vi "Teleop.vi"(0 "Call Context":T10) -> (6 "SubState 3":T1, 8 "SubState 4":T1, 9 "SubState 5":T9, 11 "Loop 3 Data":T5, 13 "Loop 4 Data":T4, 14 "SubState 0":T1=enum."driver control", 15 "Loop 1 Data":T7, 16 "Loop 0 Data":T8, 17 "SubState 1":T1, 18 "Loop 2 Data":T6, 19 "SubState 2":T1)   [LabVIEW 2013]
uses:
  typedefs/subStates.ctl
  <vilib>/Rock Robotics/WPI/DriverStation/WPI_DriverStationDerivedRobotMode.ctl
  typedefs/singleUseSubstate.ctl
  typedefs/Loop Datatypes/Loop 0 Datatype.ctl
  typedefs/Loop Datatypes/Loop 1 Datatype.ctl
  typedefs/Loop Datatypes/Loop 2 Datatype.ctl
  typedefs/Loop Datatypes/Loop 3 Datatype.ctl
  typedefs/Loop Datatypes/Loop 4 Datatype.ctl
  <vilib>/Rock Robotics/WPI/Joystick/WPI_JoystickDevRef.ctl
  <vilib>/Rock Robotics/WPI/Joystick/WPI_JoystickDeviceEnum.ctl
  typedefs/fg_typedef.ctl
  typedefs/vision enable.ctl
  <vilib>/Rock Robotics/WPI/Joystick/WPI_JoystickGetSetRefNum.vi
panel:
  out "prev lock state":T1
  out "JS3":T2
  out "Drive to DC":bool
  out "JS1":T2
  out "JS2":T2
  out "Exit Value":i32=-1
  # "Loop Data and Substates"
  # "Latch Loop"
  # "Drive Loop"
  # "Shooter Pneumatics Loop"
  # "Pickup/Passing Belts Loop"
  # "Pickup Arm Loop"
  # "Shifter Loop"
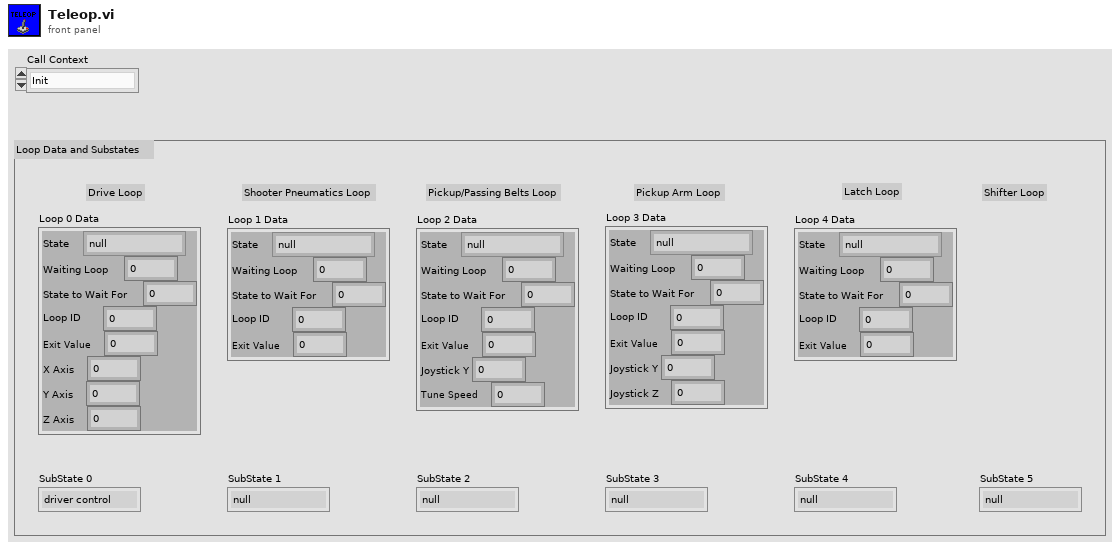
[diagram p1: front panel]
types:
  T1 = typedef "subStates.ctl" = enum16{"null", "wait", "driver control", "auto", "manual override", "hold position", "rotate", "pickup", "pass", "load", "goto shoot", "shoot", "cancel", "end"}
  T2 = typedef "WPI_JoystickDevRef.ctl" = cluster{"Device":T3}
  T3 = typedef "WPI_JoystickDeviceEnum.ctl" = enum16{"USB 1", "USB 2", "USB 3", "USB 4", "Kinect 1", "Kinect 2"}
  T4 = typedef "Loop 4 Datatype.ctl" = cluster{"State":T1, "Waiting Loop":i32, "State to Wait For":i32, "Loop ID":i32, "Exit Value":i32}
  T5 = typedef "Loop 3 Datatype.ctl" = cluster{"State":T1, "Waiting Loop":i32, "State to Wait For":i32, "Loop ID":i32, "Exit Value":i32, "Joystick Y":dbl, "Joystick Z":dbl}
  T6 = typedef "Loop 2 Datatype.ctl" = cluster{"State":T1, "Waiting Loop":i32, "State to Wait For":i32, "Loop ID":i32, "Exit Value":i32, "Joystick Y":dbl, "Tune Speed":dbl}
  T7 = typedef "Loop 1 Datatype.ctl" = cluster{"State":T1, "Waiting Loop":i32, "State to Wait For":i32, "Loop ID":i32, "Exit Value":i32}
  T8 = typedef "Loop 0 Datatype.ctl" = cluster{"State":T1, "Waiting Loop":i32, "State to Wait For":i32, "Loop ID":i32, "Exit Value":i32, "X Axis":dbl, "Y Axis":dbl, "Z Axis":dbl}
  T9 = typedef "singleUseSubstate.ctl" = enum16{"null", "wait", "shift high", "shift low"}
  T10 = typedef "WPI_DriverStationDerivedRobotMode.ctl" = enum16{"Init", "Execute", "Stop"}
  T11 = cluster{"axis 1 (x)":dbl, "axis 2 (y)":dbl, "axis 3 (throttle)":dbl, "axis 4":dbl, "axis 5":dbl, "axis 6":dbl}
  T12 = typedef "WPI_EncoderDevRef.ctl" = cluster{"DevStatus":errorcluster, "EncoderIndex":T13, "CounterIndex":T14, "DistancePerCount":dbl, "Decoding Type":T15}
  T13 = typedef "FPGA_EncoderIdx.ctl" = enum8{"Enc 0", "Enc 1", "Enc 2", "Enc 3", "Invalid"}
  T14 = typedef "FPGA_CounterCtrSystemIndex.ctl" = enum8{"Ctr 0", "Ctr 1", "Ctr 2", "Ctr 3", "Ctr 4", "Ctr 5", "Ctr 6", "Ctr 7", "Invalid"}
  T15 = typedef "WPI_EncoderType.ctl" = enum16{"1x", "2x", "4x"}
  T16 = typedef "vision enable.ctl" = enum16{"Enable", "Disable", "Stop"}
  T17 = typedef "fg_typedef.ctl" = enum16{"Get", "Set"}
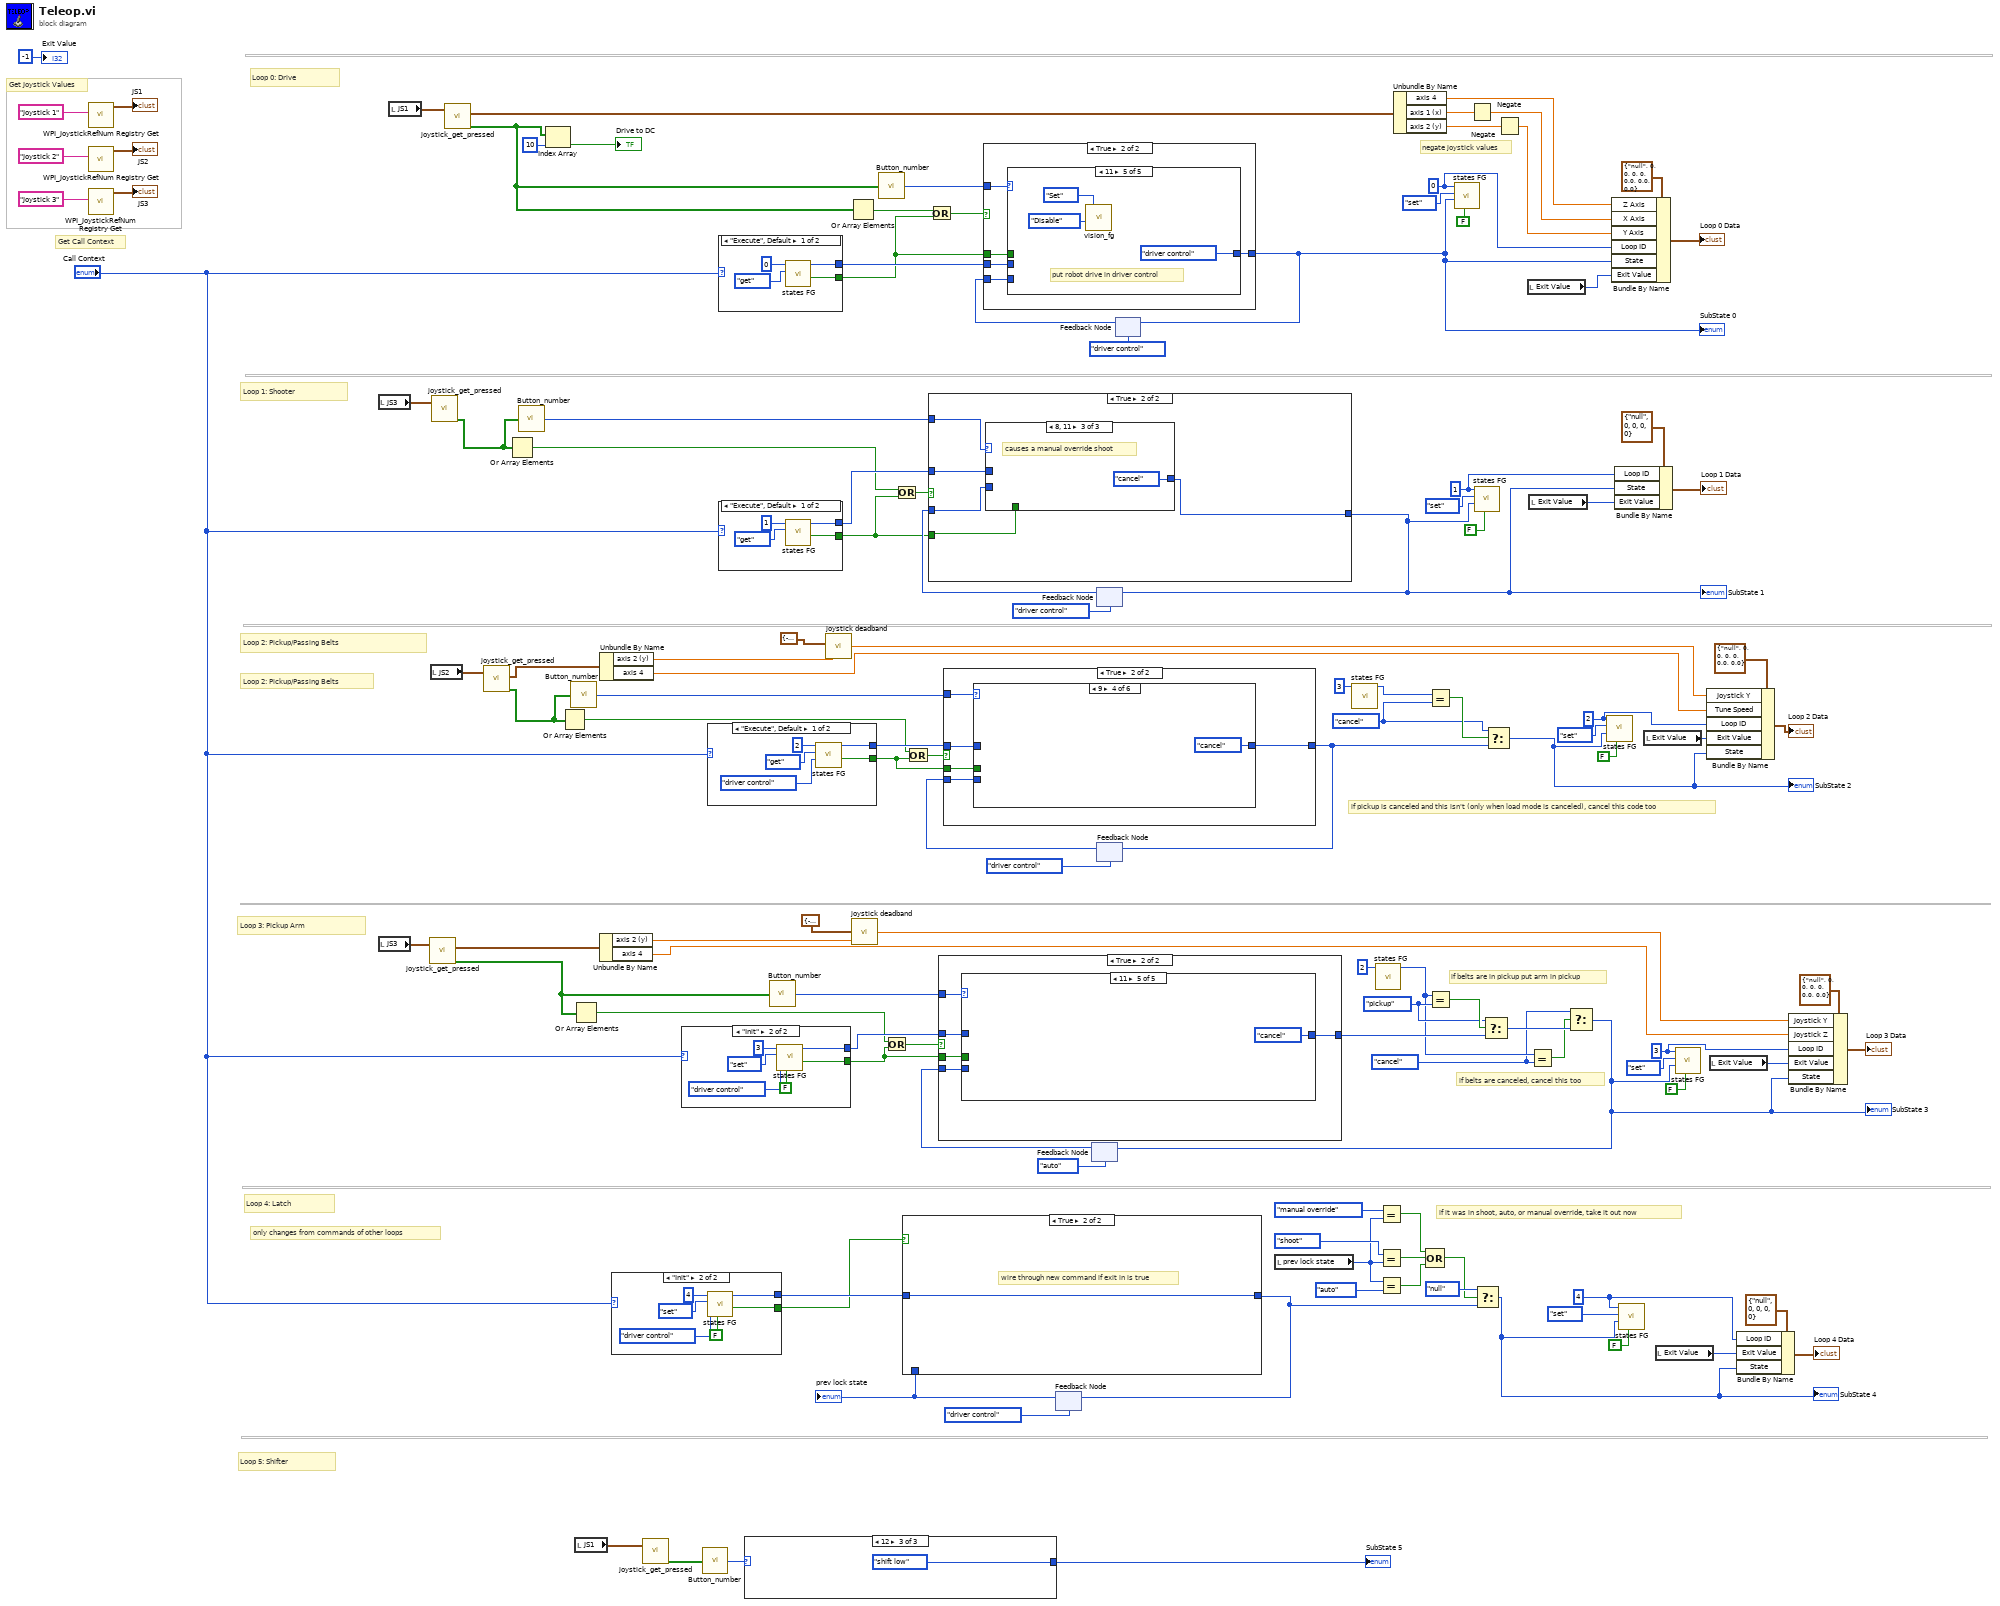
[diagram p0: block diagram]
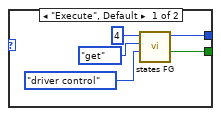
[diagram p3: hidden frame]
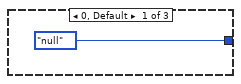
[diagram p4: hidden frame]
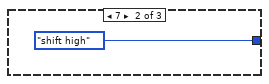
[diagram p5: hidden frame]
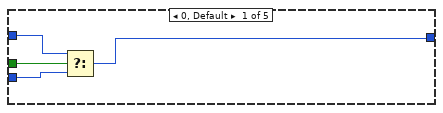
[diagram p7: hidden frame]
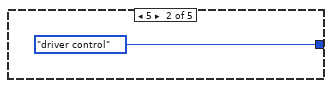
[diagram p8: hidden frame]
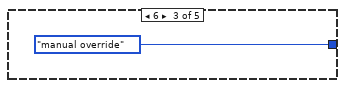
[diagram p9: hidden frame]
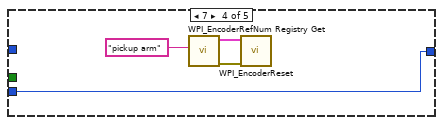
[diagram p10: hidden frame]
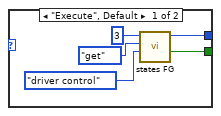
[diagram p11: hidden frame]
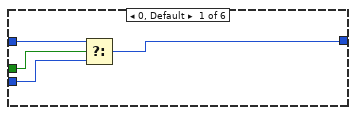
[diagram p13: hidden frame]
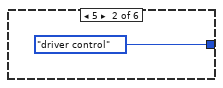
[diagram p14: hidden frame]
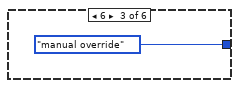
[diagram p15: hidden frame]
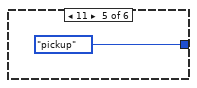
[diagram p16: hidden frame]
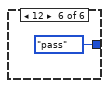
[diagram p17: hidden frame]
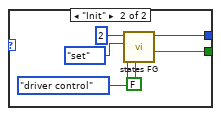
[diagram p18: hidden frame]
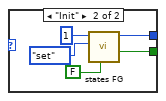
[diagram p19: hidden frame]
diagram:
  w1 = subStates."cancel" ("y")
  w8 = subStates."cancel" ("y")
  w25 = subStates."pickup" ("y")
  w36 = 4 ("Loop ID")
  w100 = 3 ("Loop ID")
  w101 = 2 ("Loop ID")
  w110 = 1 ("Loop ID")
  w112 = 0 ("Loop ID")
  # "if pickup is canceled and this isn't (only when load mode is canceled), cancel this code too"
  # "if belts are canceled, cancel this too"
  # "only changes from commands of other loops"
  # "if it was in shoot, auto, or manual override, take it out now"
  # "if belts are in pickup put arm in pickup"
  # "Loop 2: Pickup/Passing Belts"
  # "negate joystick values"
  # "Get Call Context"
  # "Get Joystick Values"
  # "Loop 4: Latch"
  # "Loop 3: Pickup Arm"
  # "Loop 5: Shifter"
  # "Loop 2: Pickup/Passing Belts"
  # "Loop 1: Shooter"
  # "Loop 0: Drive"
  n1 = call <vilib>:"WPI_JoystickRefNum Registry Get.vi"("refnum name"="Joystick 1") -> ("JoystickDevRef"=→"JS1":T2)  [unwired: 9 in, 1 out]
  n2 = call <vilib>:"WPI_JoystickRefNum Registry Get.vi"("refnum name"="Joystick 2") -> ("JoystickDevRef"=→"JS2":T2)  [unwired: 9 in, 1 out]
  n3 = call <vilib>:"WPI_JoystickRefNum Registry Get.vi"("refnum name"="Joystick 3") -> ("JoystickDevRef"=→"JS3":T2)  [unwired: 9 in, 1 out]
  n4 = local read "JS3"() -> (w77:T2)
  n5 = local read "JS3"() -> (w62:T2)
  n6 = local read "JS1"() -> (w78:T2)
  n7 = call "joystick_get_pressed.vi"("JoystickDevRef 2"=w62) -> ("Axes"=w66:T11, "Buttons Pressed?"=w43:bool[])  [unwired: 1 in, 2 out]
  n8 = local read "JS2"() -> (w50:T2)
  n9 = call "joystick_get_pressed.vi"("JoystickDevRef 2"=w77) -> ("Buttons Pressed?"=w45:bool[])  [unwired: 1 in, 3 out]
  n10 = call "joystick_get_pressed.vi"("JoystickDevRef 2"=w78) -> ("Axes"=w82:T11, "Buttons Pressed?"=w58:bool[])  [unwired: 1 in, 2 out]
  n11 = call "joystick_get_pressed.vi"("JoystickDevRef 2"=w50) -> ("Axes"=w33:T11, "Buttons Pressed?"=w34:bool[])  [unwired: 1 in, 2 out]
  n12 = Or Array Elements(Boolean array=w45) -> (logical OR=w69:bool)
  n13 = call "Button_number.vi"("Button Array"=w45) -> ("Button Pressed"=w71:i32)
  n14 = Index Array(array=w58, index=10) -> (element=→"Drive to DC":bool)
  n15 = Or Array Elements(Boolean array=w34) -> (logical OR=w49:bool)
  n16 = call "Button_number.vi"("Button Array"=w34) -> ("Button Pressed"=w48:i32)
  n17 = Or Array Elements(Boolean array=w43) -> (logical OR=w65:bool)
  n18 = local read "JS1"() -> (w53:T2)
  n19 = Unbundle By Name(w66) -> ("axis 2 (y)"=w61:dbl, "axis 4"=w29:dbl)
  n20 = Unbundle By Name(w33) -> ("axis 2 (y)"=w42:dbl, "axis 4"=w31:dbl)
  n21 = case shown="\"Init\"" "Call Context" {
    tunnel: [w131 w137] -> w13
    tunnel: [w129 w134] -> w38
    frame "Execute", Default {
      n22 = call "states FG.vi"("subState in"=subStates."driver control", "menu (get)"=enum16{"set", "get"}."get", "Loop ID"=4) -> ("exit out"=w131:bool, "subState out"=w129:T1)  [unwired: 5 in, 2 out]
    }
    frame "Init" {
      n23 = call "states FG.vi"("exit in"=FALSE, "subState in"=subStates."driver control", "menu (get)"=enum16{"set", "get"}."set", "Loop ID"=4) -> ("exit out"=w137:bool, "subState out"=w134:T1)  [unwired: 4 in, 2 out]
    }
  }
  n24 = call "joystick_get_pressed.vi"("JoystickDevRef 2"=w53) -> ("Buttons Pressed?"=w55:bool[])  [unwired: 1 in, 3 out]
  n25 = case shown="\"Init\"" "Call Context" {
    tunnel: [w142 w148] -> w63
    tunnel: [w140 w145] -> w98
    frame "Execute", Default {
      n26 = call "states FG.vi"("subState in"=subStates."driver control", "menu (get)"=enum16{"set", "get"}."get", "Loop ID"=3) -> ("exit out"=w142:bool, "subState out"=w140:T1)  [unwired: 5 in, 2 out]
    }
    frame "Init" {
      n27 = call "states FG.vi"("exit in"=FALSE, "subState in"=subStates."driver control", "menu (get)"=enum16{"set", "get"}."set", "Loop ID"=3) -> ("exit out"=w148:bool, "subState out"=w145:T1)  [unwired: 4 in, 2 out]
    }
  }
  n28 = call "Button_number.vi"("Button Array"=w55) -> ("Button Pressed"=w54:i32)
  n29 = case shown="\"Execute\", Default" "Call Context" {
    tunnel: [w153 w159] -> w68
    tunnel: [w151 w156] -> w117
    frame "Execute", Default {
      n30 = call "states FG.vi"("subState in"=subStates."driver control", "menu (get)"=enum16{"set", "get"}."get", "Loop ID"=2) -> ("exit out"=w153:bool, "subState out"=w151:T1)  [unwired: 5 in, 2 out]
    }
    frame "Init" {
      n31 = call "states FG.vi"("exit in"=FALSE, "subState in"=subStates."driver control", "menu (get)"=enum16{"set", "get"}."set", "Loop ID"=2) -> ("exit out"=w159:bool, "subState out"=w156:T1)  [unwired: 4 in, 2 out]
    }
  }
  n32 = case shown="\"Execute\", Default" "Call Context" {
    tunnel: [w163 w168] -> w75
    tunnel: [w162 w166] -> w115
    frame "Execute", Default {
      n33 = call "states FG.vi"("menu (get)"=enum16{"set", "get"}."get", "Loop ID"=0) -> ("exit out"=w163:bool, "subState out"=w162:T1)  [unwired: 6 in, 2 out]
    }
    frame "Init" {
      n34 = call "states FG.vi"("exit in"=FALSE, "menu (get)"=enum16{"set", "get"}."set", "Loop ID"=0) -> ("exit out"=w168:bool, "subState out"=w166:T1)  [unwired: 5 in, 2 out]
    }
  }
  n35 = case shown="\"Execute\", Default" "Call Context" {
    tunnel: [w172 w177] -> w72
    tunnel: [w171 w175] -> w114
    frame "Execute", Default {
      n36 = call "states FG.vi"("menu (get)"=enum16{"set", "get"}."get", "Loop ID"=1) -> ("exit out"=w172:bool, "subState out"=w171:T1)  [unwired: 6 in, 2 out]
    }
    frame "Init" {
      n37 = call "states FG.vi"("exit in"=FALSE, "menu (get)"=enum16{"set", "get"}."set", "Loop ID"=1) -> ("exit out"=w177:bool, "subState out"=w175:T1)  [unwired: 5 in, 2 out]
    }
  }
  n38 = case shown="12" w54 {
    tunnel: [singleUseSubstate."null" ("Enum") singleUseSubstate."shift high" ("Enum") singleUseSubstate."shift low" ("Enum")] -> w90
    frame 0, Default {
    }
    frame 7 {
    }
    frame 12 {
    }
  }
  "SubState 5" <- w90
  n39 = call "Button_number.vi"("Button Array"=w43) -> ("Button Pressed"=w64:i32)
  n40 = call "joystick deadband.vi"("Joystick In"=w42, "Deadband Range"=cluster{"Deadband Min":dbl, "Deadband Max":dbl} {"Deadband Min"=-0.05, "Deadband Max"=0.05}) -> ("Joystick Out"=w32:dbl)  [unwired: 4 in]
  n41 = Or Array Elements(Boolean array=w58) -> (logical OR=w76:bool)
  n42 = call "joystick deadband.vi"("Joystick In"=w61, "Deadband Range"=cluster{"Deadband Min":dbl, "Deadband Max":dbl} {"Deadband Min"=-0.05, "Deadband Max"=0.05}) -> ("Joystick Out"=w30:dbl)  [unwired: 4 in]
  n43 = call "Button_number.vi"("Button Array"=w58) -> ("Button Pressed"=w81:i32)
  n44 = Or(x=w65, y=w63) -> (x .or. y?=w67:bool)
  n45 = Or(x=w69, y=w72) -> (x .or. y?=w73:bool)
  n46 = Or(x=w49, y=w68) -> (x .or. y?=w70:bool)
  n47 = Or(x=w76, y=w75) -> (x .or. y?=w74:bool)
  n48 = feedback #1(subStates."driver control" ("Drive SubState")) -> (w12:T1)
  "prev lock state" <- w12
  n49 = case shown="True" w13 {
    tunnel: [w183 w184] -> w23
    tunnel: w38 -> [_ w184]
    tunnel: w12 -> [w183 _]
    frame False {
      # "*yawn* nothing to do...wire through the previous state"
    }
    frame True {
      # "wire through new command if exit in is true"
    }
  }
  n50 = feedback-in #1(w23) -> ()
  n51 = feedback #2(subStates."auto" ("Drive SubState")) -> (w95:T1)
  n52 = case shown="True" w67 {
    tunnel: w95 -> [w185 w186]
    tunnel: [w185 w187] -> w27
    tunnel: w98 -> [_ w188]
    tunnel: w64 -> [_ w190]
    tunnel: w63 -> [_ w189]
    frame False {
      # "boring drivers, not pressing anything...wire through the previous state"
    }
    frame True {
      n53 = case shown="11" w190 {
        tunnel: w189 -> [w194 _ _ _ _]
        tunnel: w186 -> [w193 _ _ w200 _]
        tunnel: w188 -> [w192 _ _ _ _]
        tunnel: [w191 subStates."driver control" ("Drive SubState") subStates."manual override" ("Drive SubState") w200 subStates."cancel" ("Drive SubState")] -> w187
        frame 0, Default {
          n54 = Select(t=w192, s=w194, f=w193) -> (s? t:f=w191:T1)
        }
        frame 5 {
        }
        frame 6 {
        }
        frame 7 {
          n55 = call <vilib>:"WPI_EncoderRefNum Registry Get.vi"("refnum name"="pickup arm") -> ("error out"=w198:errorcluster, "EncoderDevRef"=w197:T12)  [unwired: 9 in]
          n56 = call <vilib>:"WPI_EncoderReset.vi"("error in (no error)"=w198, "EncoderDevRef"=w197) -> ()  [unwired: 8 in, 2 out]
        }
        frame 11 {
        }
      }
    }
  }
  n57 = feedback #3(subStates."driver control" ("Drive SubState")) -> (w116:T1)
  n58 = case shown="True" w73 {
    tunnel: w116 -> [w202 w206]
    tunnel: [w202 w203] -> w83
    tunnel: w114 -> [_ w207]
    tunnel: w71 -> [_ w205]
    tunnel: w72 -> [_ w204]
    frame False {
      # "nothing pressed here, move along (wire through the previous state)"
    }
    frame True {
      n59 = case shown="8, 11" w205 {
        tunnel: w207 -> [w210 _ _]
        tunnel: w206 -> [w209 _ _]
        tunnel: [w208 subStates."load" ("Drive SubState") subStates."cancel" ("Drive SubState")] -> w203
        tunnel: w204 -> [w211 _ _]
        frame 0, Default {
          n60 = Select(t=w210, s=w211, f=w209) -> (s? t:f=w208:T1)
        }
        frame 2 {
        }
        frame 8, 11 {
          # "causes a manual override shoot"
        }
      }
    }
  }
  "SubState 1" <- w83
  n61 = feedback-in #3(w83) -> ()
  n62 = feedback #4(subStates."driver control" ("Drive SubState")) -> (w120:T1)
  n63 = case shown="True" w70 {
    tunnel: w120 -> [w214 w216]
    tunnel: [w214 w215] -> w4
    tunnel: w117 -> [_ w217]
    tunnel: w48 -> [_ w219]
    tunnel: w68 -> [_ w218]
    frame False {
      # "nothing pressed here, move along obviously and wire through the previous state"
    }
    frame True {
      n64 = case shown="9" w219 {
        tunnel: w218 -> [w223 _ _ _ _ _]
        tunnel: w217 -> [w222 _ _ _ _ _]
        tunnel: w216 -> [w221 _ _ _ _ _]
        tunnel: [w220 subStates."driver control" ("Drive SubState") subStates."manual override" ("Drive SubState") subStates."cancel" ("Drive SubState") subStates."pickup" ("Drive SubState") subStates."pass" ("Drive SubState")] -> w215
        frame 0, Default {
          n65 = Select(t=w222, s=w223, f=w221) -> (s? t:f=w220:T1)
        }
        frame 5 {
        }
        frame 6 {
        }
        frame 9 {
        }
        frame 11 {
        }
        frame 12 {
        }
      }
    }
  }
  n66 = feedback-in #4(w4) -> ()
  n67 = feedback #5(subStates."driver control" ("Drive SubState")) -> (w122:T1)
  n68 = case shown="True" w74 {
    tunnel: w122 -> [w229 w231]
    tunnel: [w229 w230] -> w52
    tunnel: w115 -> [_ w232]
    tunnel: w81 -> [_ w234]
    tunnel: w75 -> [_ w233]
    frame False {
      # "keep current state, no change necessary"
    }
    frame True {
      n69 = case shown="11" w234 {
        tunnel: w233 -> [w238 _ _ _ _]
        tunnel: w232 -> [w237 _ _ _ _]
        tunnel: w231 -> [w236 w243 w244 w252 _]
        tunnel: [w235 w239 w244 w253 subStates."driver control" ("Drive SubState")] -> w230
        frame 0, Default {
          n70 = Select(t=w237, s=w238, f=w236) -> (s? t:f=w235:T1)
        }
        frame 1 {
          w240 = subStates."hold position" ("x")
          # "button 1, hold position toggle"
          n71 = Equal?(x=w240, y=w243) -> (x = y?=w242:bool)
          n72 = Select(t=subStates."driver control" ("Drive SubState"), s=w242, f=w240) -> (s? t:f=w239:T1)
        }
        frame 8 {
          n73 = disable-structure shown="Enabled" {
            frame Disabled {
              w247 = vision_enable."Enable" ("y")
              # "toggle vision"
              n74 = call "vision_fg.vi"("Menu"=fg_typedef."Get") -> ("State Out"=w249:T16)  [unwired: 2 in, 1 out]
              n75 = Equal?(x=w249, y=w247) -> (x = y?=w248:bool)
              n76 = Select(t=vision_enable."Disable" ("y"), s=w248, f=w247) -> (s? t:f=w245:T16)
              n77 = call "vision_fg.vi"("Action"=w245, "Menu"=fg_typedef."Set") -> ()  [unwired: 1 in, 2 out]
            }
            frame Enabled {
              # "no vision at suffield"
            }
          }
        }
        frame 9 {
          n78 = disable-structure shown="Enabled" {
            disable-tunnel: [subStates."goto shoot" ("Drive SubState") w257] -> w253
            disable-tunnel: w252 -> [_ w257]
            frame Disabled {
              # "go to shoot location"
              n79 = call "vision_fg.vi"("Action"=vision_enable."Enable", "Menu"=fg_typedef."Set") -> ()  [unwired: 1 in, 2 out]
            }
            frame Enabled {
              # "no vision at suffield"
            }
          }
        }
        frame 11 {
          # "put robot drive in driver control"
          n80 = call "vision_fg.vi"("Action"=vision_enable."Disable", "Menu"=fg_typedef."Set") -> ()  [unwired: 1 in, 2 out]
        }
      }
    }
  }
  "SubState 0" <- w52
  n81 = feedback-in #5(w52) -> ()
  n82 = local read "prev lock state"() -> (w19:T1)
  n83 = call "states FG.vi"("Loop ID"=3) -> ("subState out"=w5:T1)  [unwired: 7 in, 3 out]
  n84 = call "states FG.vi"("Loop ID"=2) -> ("subState out"=w11:T1)  [unwired: 7 in, 3 out]
  n85 = Equal?(x=subStates."manual override", y=w19) -> (x = y?=w17:bool)
  n86 = Equal?(x=subStates."shoot", y=w19) -> (x = y?=w16:bool)
  n87 = Equal?(x=w19, y=subStates."auto") -> (x = y?=w15:bool)
  n88 = Unbundle By Name(w82) -> ("axis 4"=w59:dbl, "axis 1 (x)"=w87:dbl, "axis 2 (y)"=w86:dbl)
  n89 = Compound Arithmetic op=OR(w17, w16, w15) -> (w14:bool)
  n90 = Equal?(x=w5, y=w1) -> (x = y?=w3:bool)
  n91 = Equal?(x=w11, y=w25) -> (x = y?=w26:bool)
  n92 = call "states FG.vi"("exit in"=FALSE, "subState in"=w52, "menu (get)"=enum16{"set", "get"}."set", "Loop ID"=w112) -> ()  [unwired: 4 in, 4 out]
  n93 = Negate(x=w87) -> (-x=w85:dbl)
  n94 = call "states FG.vi"("exit in"=FALSE, "subState in"=w83, "menu (get)"=enum16{"set", "get"}."set", "Loop ID"=w110) -> ()  [unwired: 4 in, 4 out]
  n95 = Select(t=subStates."null", s=w14, f=w23) -> (s? t:f=w22:T1)
  "SubState 4" <- w22
  n96 = Select(t=w25, s=w26, f=w27) -> (s? t:f=w10:T1)
  n97 = Select(t=w1, s=w3, f=w4) -> (s? t:f=w2:T1)
  "SubState 2" <- w2
  n98 = Negate(x=w86) -> (-x=w84:dbl)
  n99 = local read "Exit Value"() -> (w108:i32)
  n100 = local read "Exit Value"() -> (w107:i32)
  n101 = Equal?(x=w11, y=w8) -> (x = y?=w9:bool)
  n102 = Select(t=w8, s=w9, f=w10) -> (s? t:f=w7:T1)
  "SubState 3" <- w7
  n103 = feedback-in #2(w7) -> ()
  n104 = call "states FG.vi"("exit in"=FALSE, "subState in"=w2, "menu (get)"=enum16{"set", "get"}."set", "Loop ID"=w101) -> ()  [unwired: 4 in, 4 out]
  n105 = Bundle By Name(cluster=T8 {"State"=enum."null", "Waiting Loop"=0, "State to Wait For"=0, "Loop ID"=0, "Exit Value"=0, "X Axis"=0.0, "Y Axis"=0.0, "Z Axis"=0.0} ("Cluster"), "Z Axis"=w59, "X Axis"=w85, "Y Axis"=w84, "Loop ID"=w112, "State"=w52, "Exit Value"=w108) -> (→"Loop 0 Data":T8)
  n106 = Bundle By Name(cluster=T7 {"State"=enum."null", "Waiting Loop"=0, "State to Wait For"=0, "Loop ID"=0, "Exit Value"=0} ("Cluster"), "Loop ID"=w110, "State"=w83, "Exit Value"=w107) -> (→"Loop 1 Data":T7)
  n107 = call "states FG.vi"("exit in"=FALSE, "subState in"=w22, "menu (get)"=enum16{"set", "get"}."set", "Loop ID"=w36) -> ()  [unwired: 4 in, 4 out]
  n108 = local read "Exit Value"() -> (w102:i32)
  n109 = local read "Exit Value"() -> (w37:i32)
  n110 = call "states FG.vi"("exit in"=FALSE, "subState in"=w7, "menu (get)"=enum16{"set", "get"}."set", "Loop ID"=w100) -> ()  [unwired: 4 in, 4 out]
  n111 = Bundle By Name(cluster=T6 {"State"=enum."null", "Waiting Loop"=0, "State to Wait For"=0, "Loop ID"=0, "Exit Value"=0, "Joystick Y"=0.0, "Tune Speed"=0.0} ("Loop 2 Data"), "Joystick Y"=w32, "Tune Speed"=w31, "Loop ID"=w101, "Exit Value"=w102, "State"=w2) -> (→"Loop 2 Data":T6)
  n112 = local read "Exit Value"() -> (w99:i32)
  n113 = Bundle By Name(cluster=T4 {"State"=enum."null", "Waiting Loop"=0, "State to Wait For"=0, "Loop ID"=0, "Exit Value"=0} ("Loop 4 Data"), "Loop ID"=w36, "Exit Value"=w37, "State"=w22) -> (→"Loop 4 Data":T4)
  n114 = Bundle By Name(cluster=T5 {"State"=enum."null", "Waiting Loop"=0, "State to Wait For"=0, "Loop ID"=0, "Exit Value"=0, "Joystick Y"=0.0, "Joystick Z"=0.0} ("Loop 3 Data"), "Joystick Y"=w30, "Joystick Z"=w29, "Loop ID"=w100, "Exit Value"=w99, "State"=w7) -> (→"Loop 3 Data":T5)
  "Exit Value" <- -1 ("Exit Value")
